vi "DeQueue-N.vi"(8 "error in (no error)":errorcluster, 11 "queue ref":refnum<queue>) -> (0 "error out":errorcluster, 2 "remaining States":string[](array[string]), 3 "queue out":refnum<queue>)   [LabVIEW 2022 SP3]
doc: "Use this template to build a VI to use as a subVI."
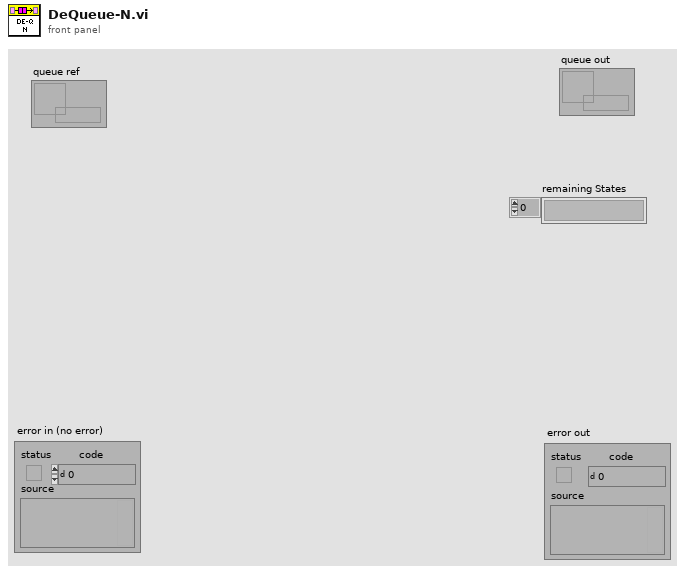
[diagram p1: front panel]
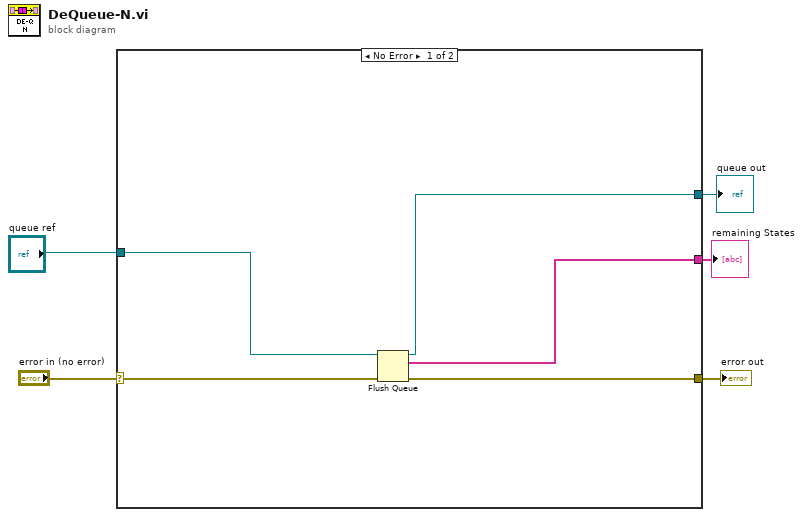
[diagram p0: block diagram]
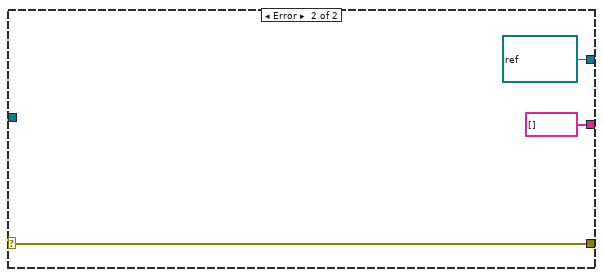
[diagram p2: hidden frame]
diagram:
  n1 = case shown="No Error" "error in (no error)" {
    selector: "error in (no error)" -> [w8 w13]
    tunnel: [w10 w13] -> w4
    tunnel: "queue ref" -> [w9 _]
    tunnel: [w7 string[] [] ("remaining elements")] -> w2
    tunnel: [w6 refnum<queue> refnum ("queue ref")] -> w1
    frame No Error {
      n2 = Flush Queue(queue=w9, error in (no error)=w8) -> (queue out=w6:refnum<queue>, remaining elements=w7:string[], error out=w10:errorcluster)
    }
    frame Error {
    }
  }
  "error out" <- w4
  "remaining States" <- w2
  "queue out" <- w1
